vi "FrameRateAdjustment.vi"(11 "FrameRate In":dbl) -> (0 "FrameInterval":dbl, 3 "FrameRate Out":dbl)   [LabVIEW 2013, in "AnimatorXControl.xctl"]
uses:
  AnimatorXControl.xctl
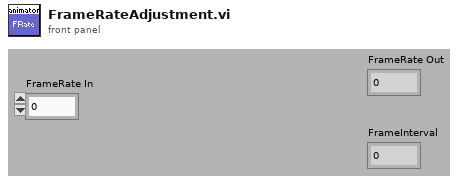
[diagram p1: front panel]
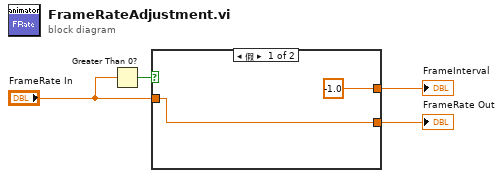
[diagram p0: block diagram]
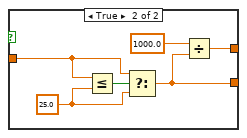
[diagram p2: hidden frame]
diagram:
  n1 = Greater Than 0?(x="FrameRate In") -> (x > 0?=w4:bool)
  n2 = case shown="假" w4 {
    tunnel: [-1.0 w9] -> w2
    tunnel: "FrameRate In" -> [w5 w8]
    tunnel: [w5 w7] -> w1
    frame False {
    }
    frame True {
      w10 = 25.0 ("y")
      n3 = Less Or Equal?(x=w8, y=w10) -> (x <= y?=w11:bool)
      n4 = Select(t=w8, s=w11, f=w10) -> (s? t:f=w7:dbl)
      n5 = Divide(x=1000.0, y=w7) -> (x/y=w9:dbl)
    }
  }
  "FrameRate Out" <- w1
  "FrameInterval" <- w2
